vi "Build Channel Cluster Array.vi"() -> (3 "Channels out":cluster{"Channels":T1[]})   [LabVIEW 2023, in "Cycler Cluster - 2 Channel.lvclass"]
uses:
  Cycler Cluster - 2 Channel.lvclass
  Utilities/Channel.ctl
  Cycler Cluster - 2 Channel.lvclass/Cycler Cluster - 2 Channel.ctl
  Utilities/Utilities.lvlib
panel:
  in  "Chiller Cluster - 2 Channel.lvclass":refnum<class "Cycler Cluster - 2 Channel.lvclass">
  in  "Channels in":cluster{"Channels":T1[]}
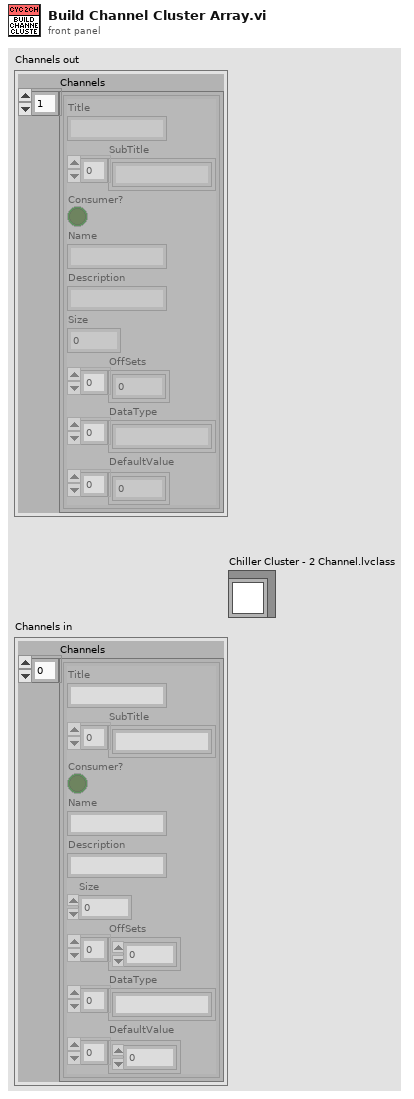
[diagram p1: front panel]
types:
  T1 = typedef "Utilities.lvlib/Channel.ctl" = cluster{"Title":string, "SubTitle":string[], "Consumer?":bool, "Name":string, "Description":string, "Size":i32, "OffSets":i32[], "DataType":string[], "DefaultValue":dbl[]}
  T2 = cluster{"OnOff.ACT":bool, "ErrorAcknowledge.ACT":bool, "IsoMeasurement.ACT":bool, "ParallelMode.ACT":bool}
  T3 = cluster{"OnOff.STS":i32, "Error.STS":i32, "Watchdog.STS":i32, "IsoMeasurement.STS":i32, "ParallelMode.STS":i32}
  T4 = cluster{"ErrorAcknowledge.ch01.ACT":bool, "OutputEnable.ch01.ACT":bool, "ControlMode.ch01.CTL":u16, "Voltage.ch01.SP":dbl, "VoltageMIN.ch01.SP":dbl, "VoltageMAX.ch01.SP":dbl, "VoltageGrad.ch01.SP":dbl, "Current.ch01.SP":dbl, "CurrentMIN.ch01.SP":dbl, "CurrentMAX.ch01.SP":dbl, "CurrentGrad.ch01.SP":dbl, "Power.ch01.SP":dbl, "Power.ch01.SP":dbl, "Power.ch01.SP":dbl, "PowerGrad.ch01.SP":dbl, "ParameterSet.ch01.CTL":i32}
  T5 = cluster{"Error.ch01.STS":i32, "OutputEnable.ch01.STS":i32, "ControlMode.ch01.STS":u16, "Voltage.ch01.AV":dbl, "Current.ch01.AV":dbl, "Power.ch01.AV":dbl, "VoltageNominal.ch01.AV":dbl, "CurrentNominal.ch01.AV":dbl, "PowerNominal.ch01.AV":dbl, "ParameterSet.ch01.STS":i32}
  T6 = cluster{"ErrorAcknowledge.ch02.ACT":bool, "OutputEnable.ch02.ACT":bool, "ControlMode.ch02.CTL":u16, "Voltage.ch02.SP":dbl, "VoltageMIN.ch02.SP":dbl, "VoltageMAX.ch02.SP":dbl, "VoltageGrad.ch02.SP":dbl, "Current.ch02.SP":dbl, "CurrentMIN.ch02.SP":dbl, "CurrentMAX.ch02.SP":dbl, "CurrentGrad.ch02.SP":dbl, "Power.ch02.SP":dbl, "PowerMIN.ch02.SP":dbl, "PowerMAX.ch02.SP":dbl, "PowerGrad.ch02.SP":dbl, "ParameterSet.ch02.CTL":i32}
  T7 = cluster{"Error.ch02.STS":i32, "OutputEnable.ch02.STS":i32, "ControlMode.ch02.STS":u16, "Voltage.ch02.AV":dbl, "Current.ch02.AV":dbl, "Power.ch02.AV":dbl, "VoltageNominal.ch02.AV":dbl, "CurrentNominal.ch02.AV":dbl, "PowerNominal.ch02.AV":dbl, "ParameterSet.ch02.STS":i32}
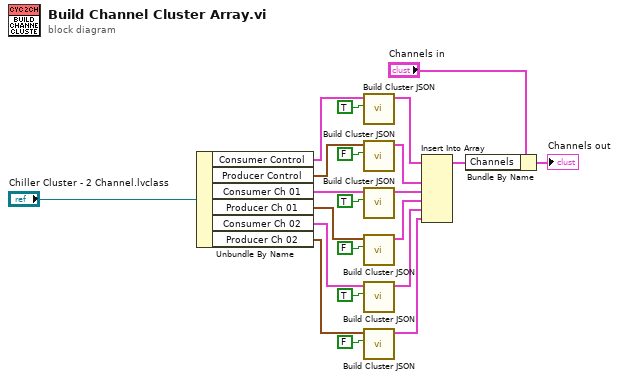
[diagram p0: block diagram]
diagram:
  n1 = Unbundle By Name("Chiller Cluster - 2 Channel.lvclass") -> ("Consumer Control"=w22:T2, "Producer Control"=w21:T3, "Consumer Ch 01"=w10:T4, "Producer Ch 01"=w11:T5, "Consumer Ch 02"=w2:T6, "Producer Ch 02"=w1:T7)
  n2 = call "Build Cluster JSON.vi"("Consumer?"=TRUE, "Cluster"=w22) -> ("Array"=w18:T1[])  [unwired: 9 in]
  n3 = call "Build Cluster JSON.vi"("Consumer?"=FALSE, "Cluster"=w21) -> ("Array"=w17:T1[])  [unwired: 9 in]
  n4 = call "Build Cluster JSON.vi"("Consumer?"=TRUE, "Cluster"=w10) -> ("Array"=w9:T1[])  [unwired: 9 in]
  n5 = call "Build Cluster JSON.vi"("Consumer?"=FALSE, "Cluster"=w11) -> ("Array"=w8:T1[])  [unwired: 9 in]
  n6 = call "Build Cluster JSON.vi"("Consumer?"=TRUE, "Cluster"=w2) -> ("Array"=w4:T1[])  [unwired: 9 in]
  n7 = call "Build Cluster JSON.vi"("Consumer?"=FALSE, "Cluster"=w1) -> ("Array"=w3:T1[])  [unwired: 9 in]
  n8 = Insert Into Array(array=w18, new element #1=w17, new element #2=w9, new element #3=w8, new element #4=w4, new element #5=w3) -> (w15:T1[])  [unwired: 1 in]
  n9 = Bundle By Name(cluster="Channels in", "Channels"=w15) -> (→"Channels out":cluster{"Channels":T1[]})
